vi "sub_Gslam.vi"(10 "hz":dbl[][][](array[numeric]), 11 "hxDR":cluster{"x":dbl, "y":dbl, "yaw":dbl}[](array[cluster])) -> ()   [LabVIEW 2019]
uses:
  <vilib>/Analysis/Matrix/Datatypes/RealMatrix.ctl
  Ctrl/cmd_common.ctl
  <vilib>/Analysis/Matrix/Numeric/Conversions/Array To Matrix - RA2.vi
  <vilib>/Analysis/Matrix/Numeric/Conversions/Array To Matrix - RA.vi
  <vilib>/Analysis/Matrix/Numeric/Add/Add - RM,RM.vi
  <vilib>/imath/engines/lvmath2/RunTimeEngine/Managers/WorkSpace/UID Generator.vi
  <vilib>/Analysis/Matrix/Numeric/Conversions/Matrix To Array - RM.vi
  <vilib>/imath/engines/lvmath2/RunTimeEngine/BuiltInFunctions/inv/NIMS_inv(GM).vi
  <instcachedir>/0/NIMS_inv(GM)_A6DF8FE880224208AACFE4CF9F659502.lvgen/NIMS_inv(GM)_A6DF8FE880224208AACFE4CF9F659502_000.vi
  <vilib>/imath/engines/lvmath2/RunTimeEngine/RunTimeType/NIMS_RunTimeType_From StrictType (excl LVString).vi
  <instcachedir>/0/NIMS_RunTimeType_From StrictType (excl LVString)_D8AFBA86A94845AAA577C895450664BD.lvgen/NIMS_RunTimeType_From StrictType (excl LVString)_D8AFBA86A94845AAA577C895450664BD_000.vi
  <vilib>/imath/engines/lvmath2/RunTimeEngine/ErrorHandling/NIMS_Error From Error Code.vi
  <vilib>/imath/engines/lvmath2/RunTimeEngine/LocalVariableDefStatement/MC_LocalVariableDefStatement_Display.vi
  <vilib>/imath/engines/lvmath2/RunTimeEngine/Managers/SymbolTable/Clear UID.vi
  <vilib>/imath/engines/lvmath2/RunTimeEngine/NodeEndStatement/NIMS_NodeEndStatement_Output.vi
  <instcachedir>/0/NIMS_NodeEndStatement_Output_53EC0D466D134D7ABD903AC30B43404B.lvgen/NIMS_NodeEndStatement_Output_53EC0D466D134D7ABD903AC30B43404B_002.vi
  <vilib>/imath/engines/lvmath2/RunTimeEngine/ErrorHandling/NIMS_Finalize Error.vi
  <vilib>/Analysis/baseanly.llb/Real Inverse Matrix.vi
  <vilib>/Analysis/Matrix/Numeric/Multiply/Multiply - RM,RM.vi
  <vilib>/Analysis/Matrix/NI_Matrix.lvlib
  <vilib>/Analysis/NI_AALBase.lvlib
  <vilib>/imath/engines/lvmath2/RunTimeEngine/Managers/SymbolTable/NIMS_WorkSpace.lvlib
panel:
  out "H out":T1 caption="H"
  out "i2":i32
  out "B":dbl[][](array[numeric])
  out "열의 개수":i32
  out "출력 행렬":T1
  out "error":i32 caption="에러"
  out "-x":T1
  out "원소":dbl
  out "i1":i32
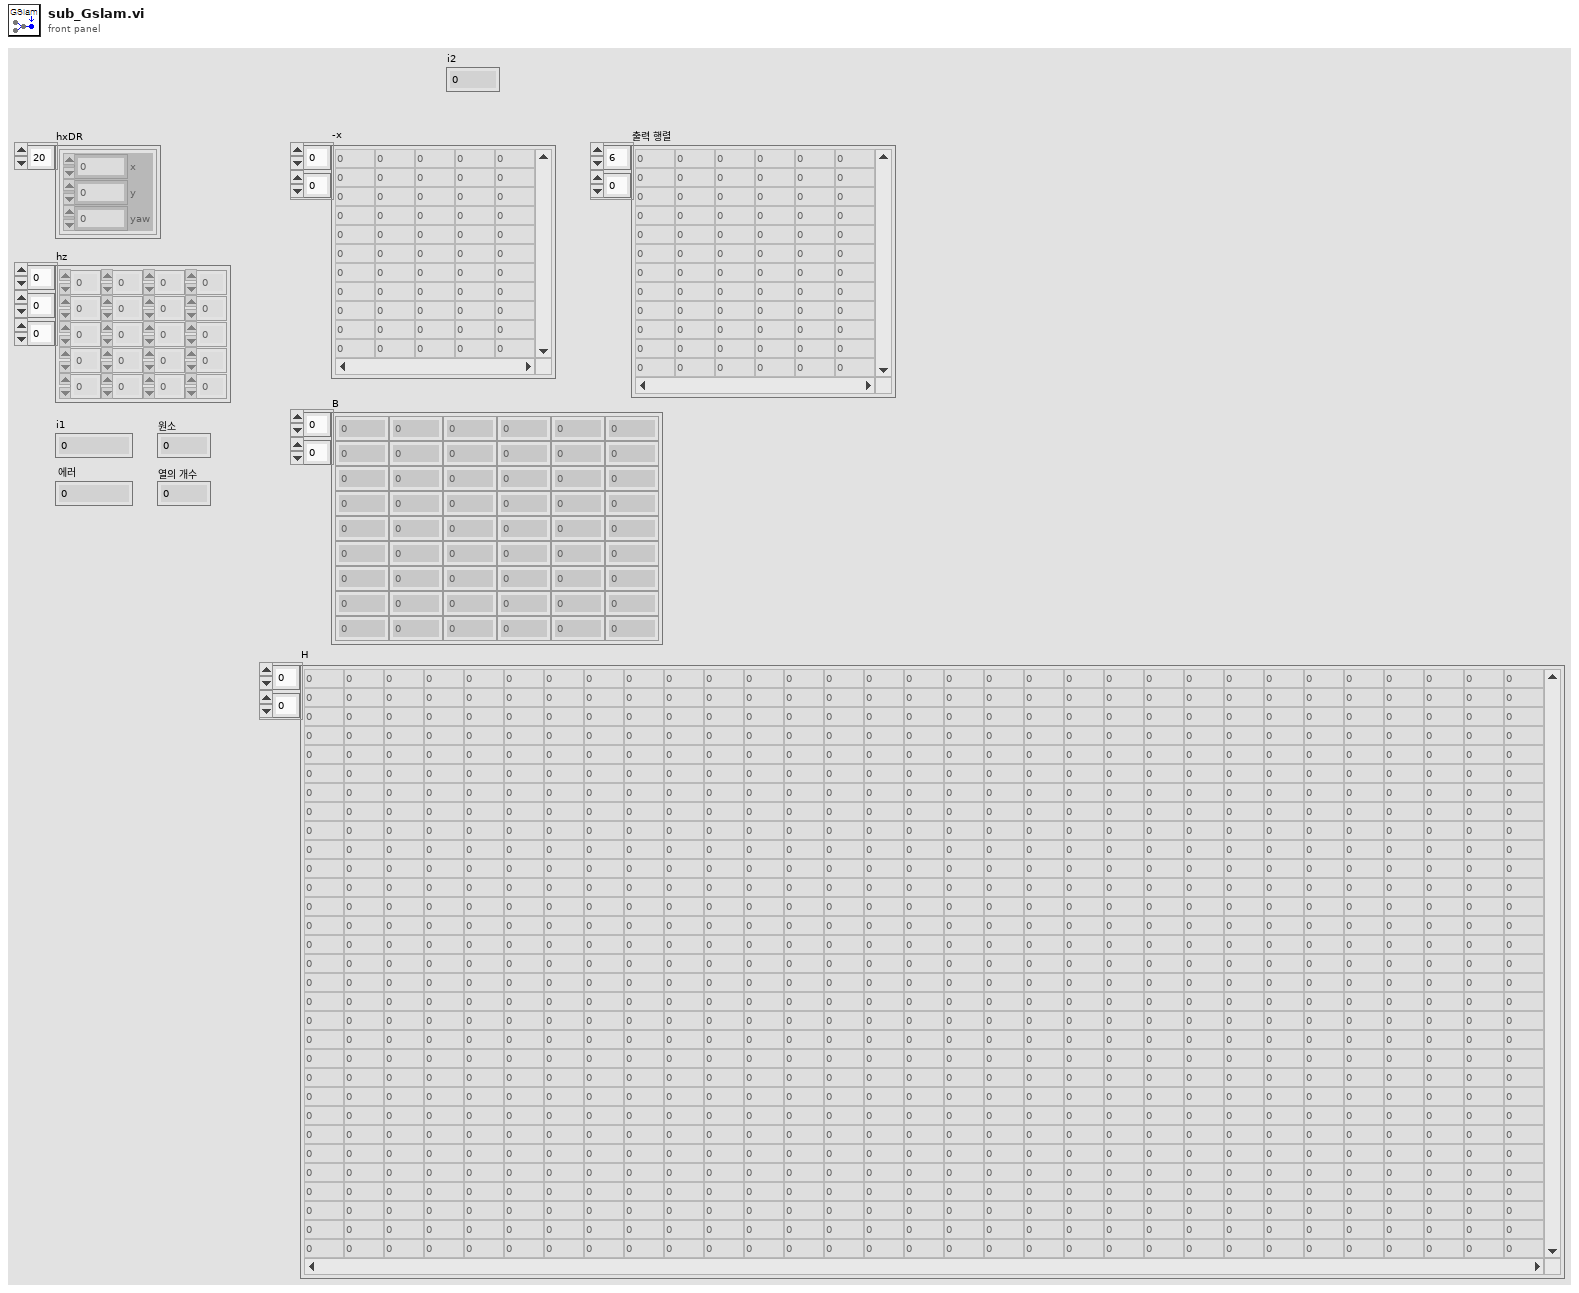
[diagram p1: front panel]
types:
  T1 = typedef "NI_Matrix.lvlib/RealMatrix.ctl" = dbl[][]
  T2 = typedef "cmd_common.ctl" = enum16{"read", "write"}
  T3 = cluster{"Q Sim":T1, "R Sim":T1, "DT":dbl, "SIM_TIME":dbl, "MAX_RANGE":dbl, "STATE_SIZE":i32, "C_SIGMA 1":dbl, "C_SIGMA 2":dbl, "C_SIGMA 3":dbl, "MAX_ITR":u32}
  T4 = cluster{"e":T1, "omega":T1, "d1":dbl, "d2":dbl, "yaw1":dbl, "yaw2":dbl, "angle1":dbl, "angle2":dbl, "id1":i32, "id2":i32}[]
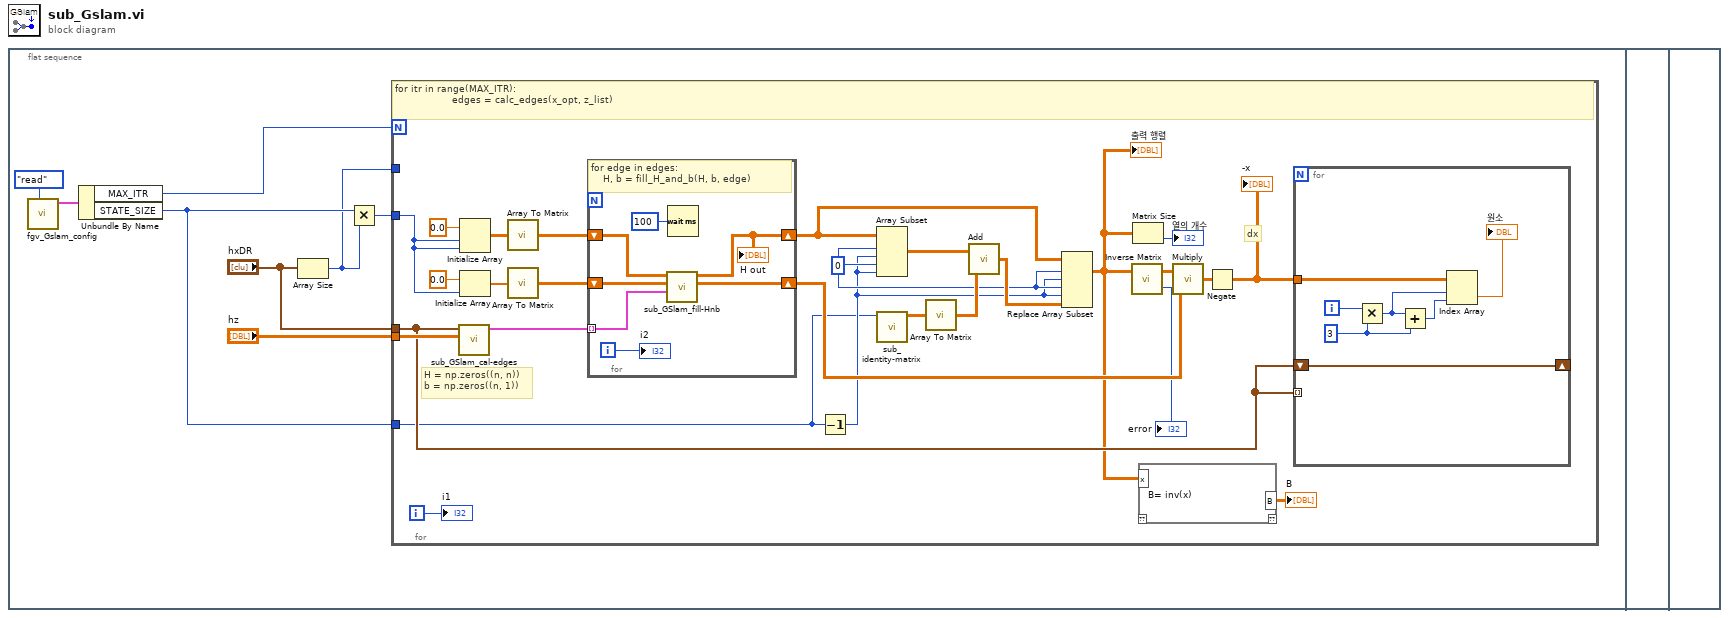
[diagram p0: block diagram]
diagram:
  n1 = flat-sequence {
    frame #0 {
      n2 = call "fgv_Gslam_config.vi"("cmd"=cmd_common."read") -> ("G cofnig out"=w7:T3)  [unwired: 10 in]
      n3 = Unbundle By Name(w7) -> ("MAX_ITR"=w5:u32, "STATE_SIZE"=w2:i32)
      n4 = Array Size(array="hxDR") -> (size(s)=w1:i32)
      n5 = Multiply(x=w2, y=w1) -> (x*y=w4:i32)
      n6 = for {
        N: w5 -> [_]
        tunnel: "hz" -> [w35]
        tunnel: "hxDR" -> [w16]
        tunnel: w4 -> [w31]
        tunnel: w2 -> [w13]
        tunnel: w1 -> [_]
        i -> [w34]
        w20 = 0 ("행 1")
        # "dx"
        # "H = np.zeros((n, n))\nb = np.zeros((n, 1))"
        # "for itr in range(MAX_ITR):\n                   edges = calc_edges(x_opt, z_list)"
        n7 = call "sub_GSlam_cal-edges.vi"("z_list"=w35, "x_list"=w16) -> ("edge arr"=w28:T4)  [unwired: 8 in, 1 out]
        n8 = Initialize Array(0.0 ("원소"), w31, w31) -> (w30:dbl[][])
        n9 = Initialize Array(0.0 ("원소"), w31) -> (w29:dbl[])
        n10 = call-poly <vilib>:"Array To Matrix.vi"("Real 2D Array"=w30) -> ("Real Matrix"=w27:T1)
        n11 = call-poly <vilib>:"Array To Matrix.vi"("Real 1D Array"=w29) -> ("Real Matrix (Column Vector)"=w26:T1)
        n12 = for {
          tunnel: w28 -> [w92] mode=indexing
          shift-right: [w91] -> w22
          shift-left: w27 -> [w94]
          shift-right: [w90] -> w17
          shift-left: w26 -> [w93]
          i -> [w89]
          # "for edge in edges:\n    H, b = fill_H_and_b(H, b, edge)"
          n13 = call "sub_GSlam_fill-Hnb.vi"("edge"=w92, "b"=w93, "H"=w94) -> ("b out"=w90:T1, "H out"=w91:T1)  [unwired: 7 in]
          "H out" <- w91
          n14 = Wait (ms)(milliseconds to wait=u32 100 ("대기 시간 (ms)")) -> ()  [unwired: 1 out]
          "i2" <- w89
        }
        n15 = Decrement(x=w13) -> (x-1=w14:i32)
        n16 = Array Subset(array=w22, index (row)=w20, length (row)=w14, index (col)=w20, length (col)=w14) -> (w25:T1)
        n17 = call "sub_identity-matrix.vi"("STATE_SIZE"=w13) -> ("identity"=w24:dbl[][])  [unwired: 10 in]
        n18 = call-poly <vilib>:"Array To Matrix.vi"("Real 2D Array"=w24) -> ("Real Matrix"=w23:T1)
        n19 = call-poly <vilib>:"Add.vi"("Real Matrix B"=w23, "Real Matrix A"=w25) -> ("A + B"=w21:T1)
        n20 = Replace Array Subset(array=w22, new element=w21, index (dim 0)=w20, index (dim 1)=w14, index (dim 2)=w20, index (dim 3)=w14) -> (w10:T1)
        "출력 행렬" <- w10
        n21 = call-poly <vilib>:"Inverse Matrix.vi"("Input Matrix"=w10) -> ("error"=→"error":i32, "Inverse Matrix"=w18:T1)  [unwired: 1 in]
        n22 = Matrix Size(0:w10) -> (2:→"열의 개수":i32)  [unwired: 1 out]
        n23 = mathscript code="B= inv(x)"("x"=w10) -> ("B"=→"B":dbl[][])  [unwired: 1 in, 1 out]
        n24 = call-poly <vilib>:"Multiply.vi"("Real Matrix B"=w17, "Real Matrix A"=w18) -> ("A * B"=w19:T1)
        n25 = Negate(x=w19) -> (-x=w15:T1)
        "-x" <- w15
        n26 = for {
          shift-right: [w82] -> _
          shift-left: w16 -> [w82]
          tunnel: w16 -> [_] mode=indexing
          tunnel: w15 -> [w87]
          i -> [w86]
          w83 = 3 ("y")
          n27 = Multiply(x=w86, y=w83) -> (x*y=w85:i32)
          n28 = Add(x=w85, y=w83) -> (x+y=w84:i32)
          n29 = Index Array(array=w87, index (row)=w85, index (col)=w84) -> (element=→"원소":dbl)
        }
        "i1" <- w34
      }
    }
    frame #1 {
    }
    frame #2 {
    }
  }
